vi "Set_Gain_DHPVA_Series.vi"(3 "error in":errorcluster, 4 "Status":i32, 5 "Gain [dB]":T1(ring), 6 "index":i32) -> (0 "error out":errorcluster, 1 "Status_out":i32, 2 "index_out":i32)   [LabVIEW 2010, in "FEMTO_LUCI-10.lvlib"]
uses:
  <userlib>/FEMTO/FEMTO_LUCI-10.lvlib
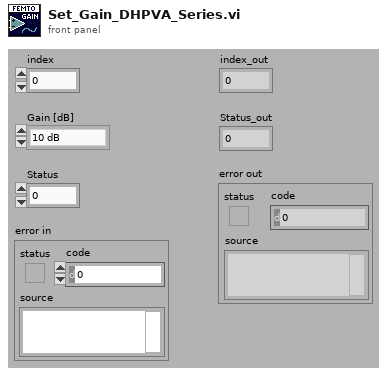
[diagram p1: front panel]
types:
  T1 = enum16{"10 dB", "20 dB", "30 dB", "40 dB", "50 dB", "60 dB"}
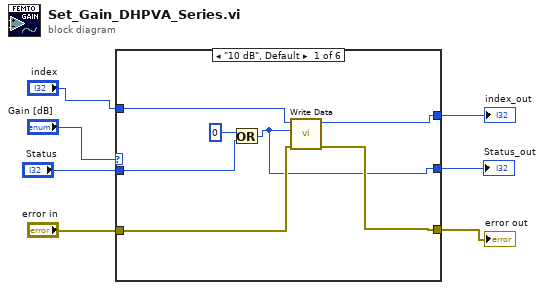
[diagram p0: block diagram]
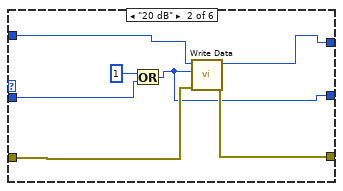
[diagram p2: hidden frame]
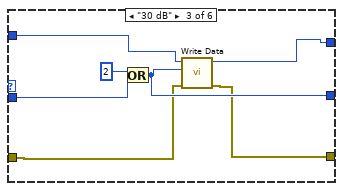
[diagram p3: hidden frame]
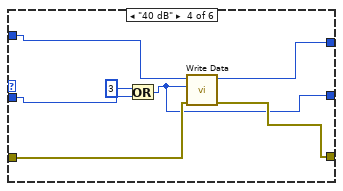
[diagram p4: hidden frame]
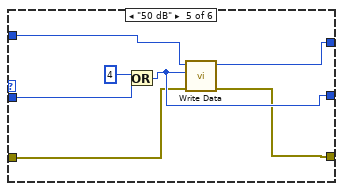
[diagram p5: hidden frame]
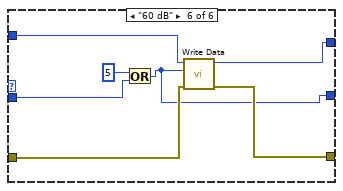
[diagram p6: hidden frame]
diagram:
  n1 = case shown="\"10 dB\", Default" "Gain [dB]" {
    tunnel: "index" -> [w13 w21 w27 w34 w41 w48]
    tunnel: [w12 w20 w26 w33 w40 w47] -> w2
    tunnel: "error in" -> [w10 w19 w23 w31 w38 w45]
    tunnel: [w9 w18 w24 w30 w36 w44] -> w4
    tunnel: "Status" -> [w11 w17 w22 w32 w37 w46]
    tunnel: [w8 w16 w25 w29 w39 w43] -> w6
    frame "10 dB", Default {
      n2 = Or(x=0 ("data_low"), y=w11) -> (x .or. y?=w8:i32)
      n3 = call <userlib>:"Write Data.vi"("error in (no error)"=w10, "data_low"=w8, "index"=w13) -> ("error out"=w9:errorcluster, "index_out"=w12:i32)  [unwired: 1 in, 6 out]
    }
    frame "20 dB" {
      n4 = Or(x=1 ("data_low"), y=w17) -> (x .or. y?=w16:i32)
      n5 = call <userlib>:"Write Data.vi"("error in (no error)"=w19, "data_low"=w16, "index"=w21) -> ("error out"=w18:errorcluster, "index_out"=w20:i32)  [unwired: 1 in, 6 out]
    }
    frame "30 dB" {
      n6 = Or(x=2 ("data_low"), y=w22) -> (x .or. y?=w25:i32)
      n7 = call <userlib>:"Write Data.vi"("error in (no error)"=w23, "data_low"=w25, "index"=w27) -> ("error out"=w24:errorcluster, "index_out"=w26:i32)  [unwired: 1 in, 6 out]
    }
    frame "40 dB" {
      n8 = Or(x=3 ("data_low"), y=w32) -> (x .or. y?=w29:i32)
      n9 = call <userlib>:"Write Data.vi"("error in (no error)"=w31, "data_low"=w29, "index"=w34) -> ("error out"=w30:errorcluster, "index_out"=w33:i32)  [unwired: 1 in, 6 out]
    }
    frame "50 dB" {
      n10 = Or(x=4 ("data_low"), y=w37) -> (x .or. y?=w39:i32)
      n11 = call <userlib>:"Write Data.vi"("error in (no error)"=w38, "data_low"=w39, "index"=w41) -> ("error out"=w36:errorcluster, "index_out"=w40:i32)  [unwired: 1 in, 6 out]
    }
    frame "60 dB" {
      n12 = Or(x=5 ("data_low"), y=w46) -> (x .or. y?=w43:i32)
      n13 = call <userlib>:"Write Data.vi"("error in (no error)"=w45, "data_low"=w43, "index"=w48) -> ("error out"=w44:errorcluster, "index_out"=w47:i32)  [unwired: 1 in, 6 out]
    }
  }
  "index_out" <- w2
  "error out" <- w4
  "Status_out" <- w6
